vi "pp_saveStimList.vi"(4 "error in (no error)":errorcluster, 6 "Path In":path, 7 "Stimulus List":dbl[][](array[numeric])) -> (0 "error out":errorcluster, 2 "Path":path)   [LabVIEW 2013]
uses:
  <vilib>/Utility/file.llb/Write To Spreadsheet File (DBL).vi
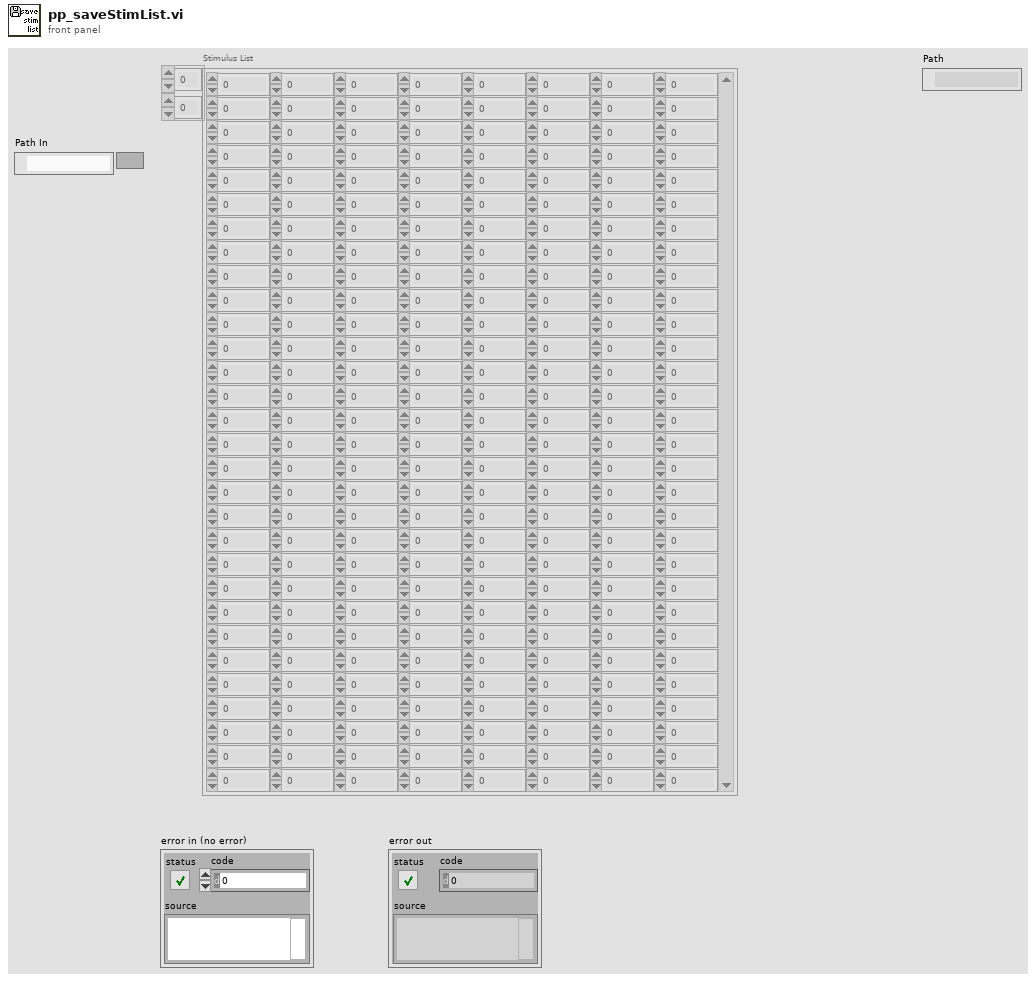
[diagram p1: front panel]
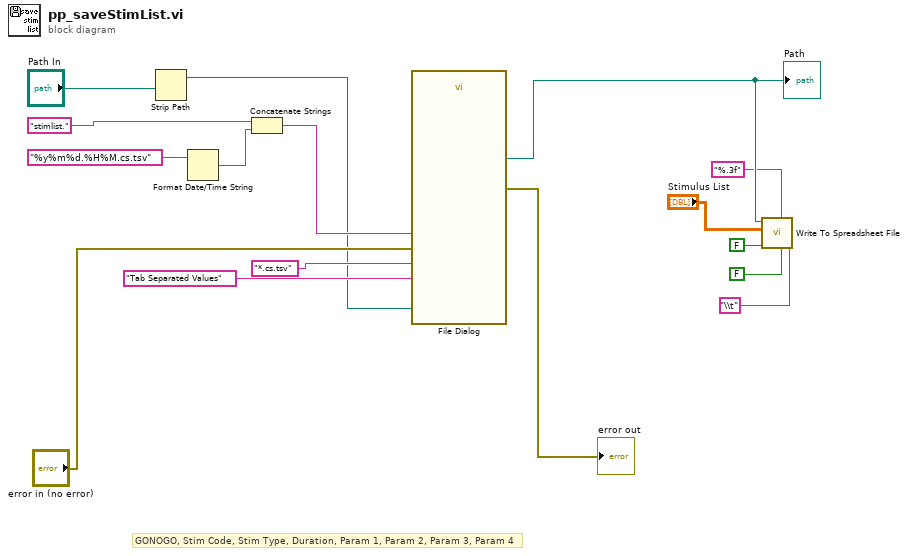
[diagram p0: block diagram]
diagram:
  # "GONOGO, Stim Code, Stim Type, Duration, Param 1, Param 2, Param 3, Param 4"
  n1 = Strip Path(path="Path In") -> (stripped path=w2:path)  [unwired: 1 out]
  n2 = Format Date/Time String(time format string (%c)="%y%m%d.%H%M.cs.tsv") -> (date/time string=w6:string)  [unwired: 2 in]
  n3 = Concatenate Strings("stimlist.", w6) -> (w5:string)
  n4 = call "File Dialog"("start path"=w2, "default name"=w5, "error in"="error in (no error)", "pattern (all files)"="*.cs.tsv", "pattern label"="Tab Separated Values") -> ("selected path"=w11:path, "error out"=→"error out":errorcluster)  [unwired: 7 in, 2 out]
  "Path" <- w11
  n5 = call-poly <vilib>:"Write To Spreadsheet File.vi"("delimiter (\\t)"="\\t" ("delimiter (\\t)"), "transpose? (no:F)"=FALSE, "format (%.3f)"="%.3f", "append to file? (new file:F)"=FALSE, "2D data"="Stimulus List", "file path (dialog if empty)"=w11) -> ()  [unwired: 2 in, 1 out]
